vi "XImc Example One axis.vi"() -> ()   [LabVIEW 2012]
uses:
  subvi/XImc Example 1 CS.ctl
  libximc.lvlib
panel:
  in  "?":enum32{"Move settings"}(tab)
  in  "Speed":i32
  in  "GMOV":bool
  in  "SMOV":bool
  in  "Accel":i32
  in  "Decel":i32
  in  "Antiplay":i32
  out "Speed":dbl format="%#.2f"
  out "Accel":i16
  out "Decel":i16 format="%#.2f"
  out "Antiplay":i32
  out "Speed":dbl format="%#.2f steps/s"
  out "Temperature":dbl format="%#.2f C"
  out "USB current":dbl format="%#.2f mA"
  out "USB voltage":dbl format="%#.2f V"
  out "Power current":dbl format="%#.2f mA"
  out "Power voltage":dbl format="%#.2f V"
  in  "Stop motion":bool
  in  "ZEROCOMM":bool
  in  "HOME":bool
  in  "RIGHT":bool
  in  "LEFT":bool
  out "controller serial number":u32
  out "function return":i32
  out "Id":i32
  in  "SSTP":bool
  in  "Shift on":bool
  in  "?":i32
  in  "Move to":bool
  in  "?":i32
  out "?":dbl format="%#.2f"
  in  "Controller":u16(ring) items=["\\\\.\\COM7"]
  in  "Find controllers":bool
  in  "Close application":bool
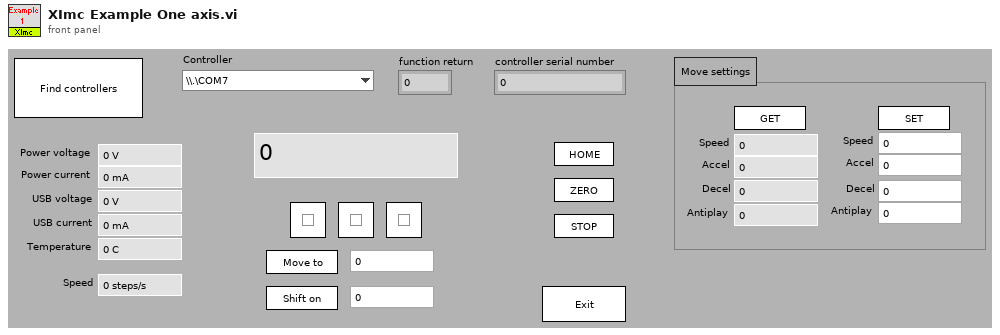
[diagram p1: front panel]
types:
  T1 = typedef "XImc Example 1 CS.ctl" = enum16{"Initialize_App", "Idle", "Find_Controllers", "Initialize_Controller", "Set_Parameters", "Get_Status", "Start_Motion", "Move_Relative", "Stop_Motion", "ZEROCOMM", "HOME", "LEFT", "RIGT", "SSTP", "Close_Controller", "Error_Handler", "Close_App", "Get_Move_Settings", "Set_Move_Settings"}
  T2 = cluster{"enumeration":i32, "Number of controllers":i32, "Controller name":string[], "variant":variant, "quit":bool, "Id":i32}
  T3 = cluster{"MoveSts":u32, "MvCmdSts":u32, "PWRSts":u32, "EncSts":u32, "WindSts":u32, "CurPosition":i32, "uCurPosition":i32, "@dummy control@":i8, "@dummy control@":i8, "@dummy control@":i8, "@dummy control@":i8, "EncPosition":i64, "CurSpeed":i32, "uCurSpeed":i32, "Ipwr":i32, "Upwr":i32, "Iusb":i32, "Uusb":i32, "CurT":i32, "Flags":u32, "GPIOFlags":u32, "CmdBufFreeSpace":u32}
  T4 = cluster{"Speed":u32, "uSpeed":u32, "Accel":u32, "Decel":u32, "AntiplaySpeed":u32, "uAntiplaySpeed":u32}
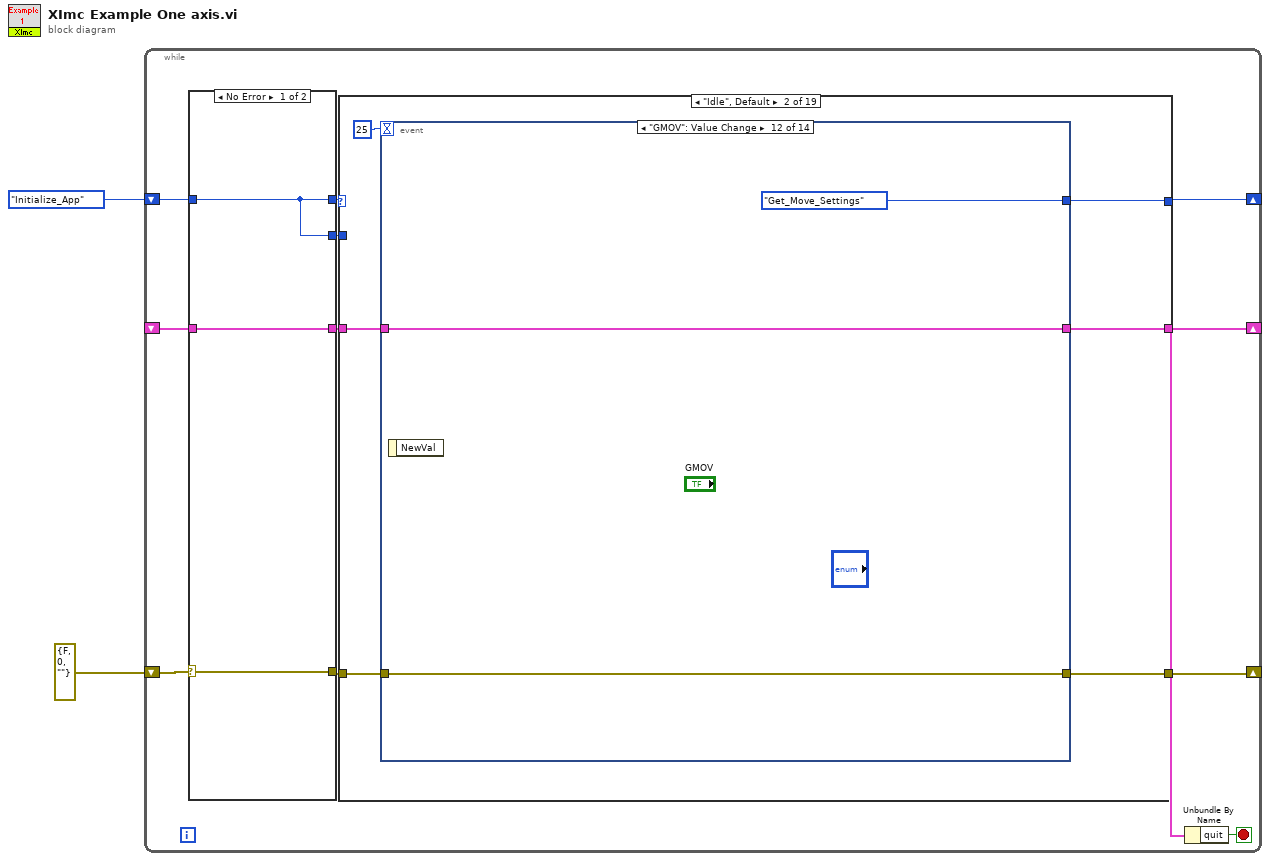
[diagram p0: block diagram]
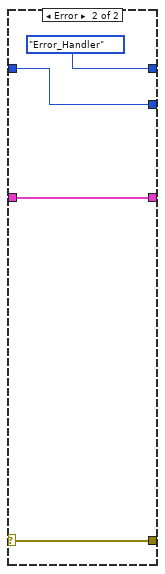
[diagram p2: hidden frame]
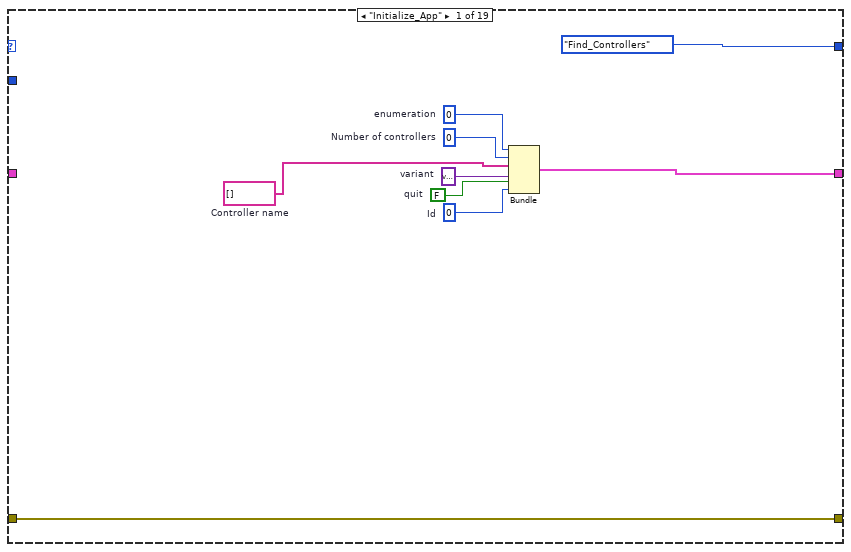
[diagram p3: hidden frame]
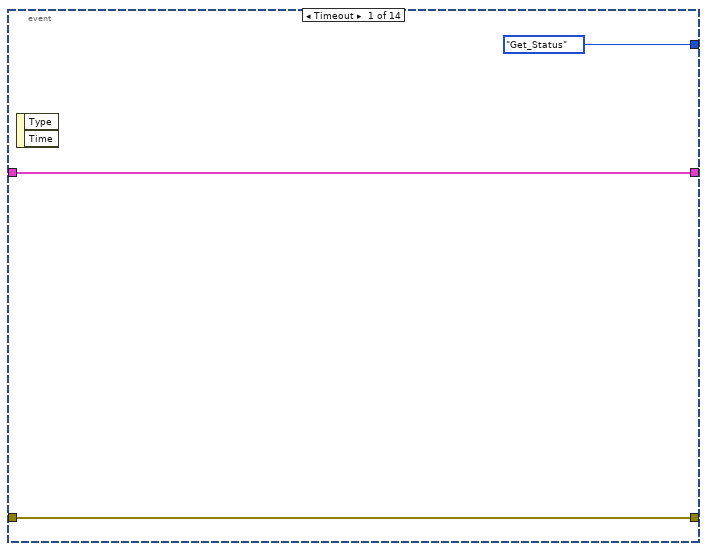
[diagram p4: hidden frame]
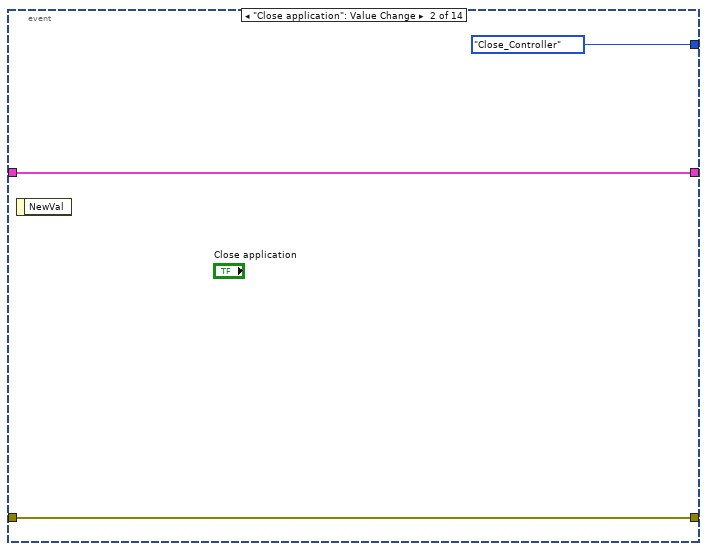
[diagram p5: hidden frame]
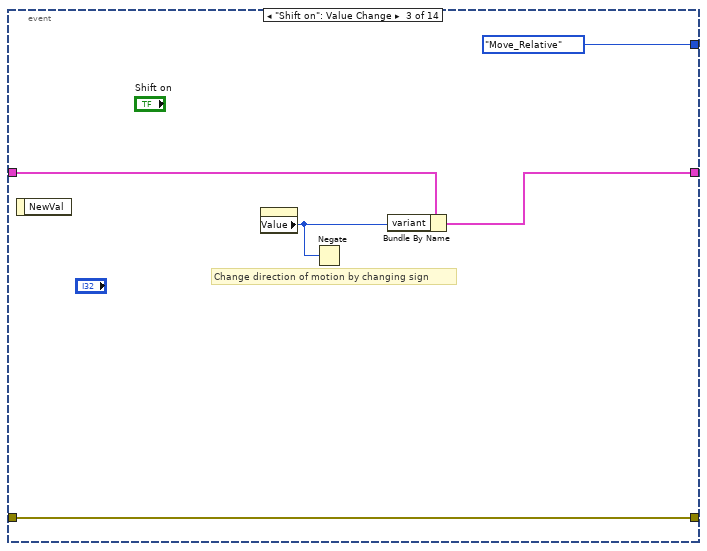
[diagram p6: hidden frame]
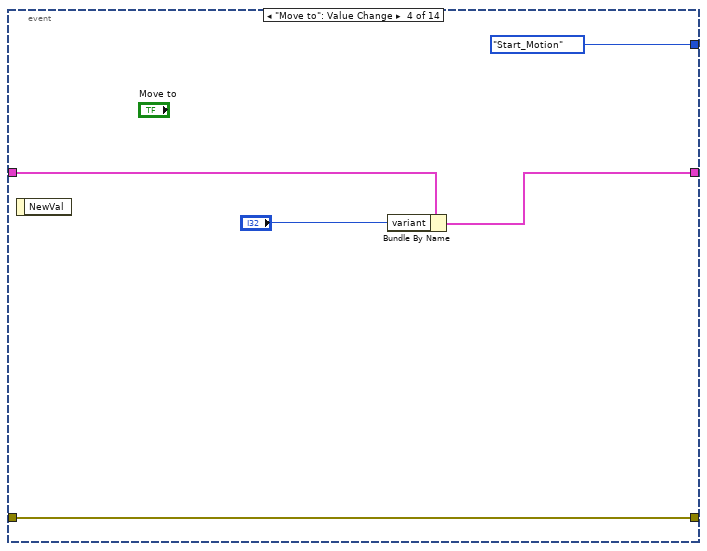
[diagram p7: hidden frame]
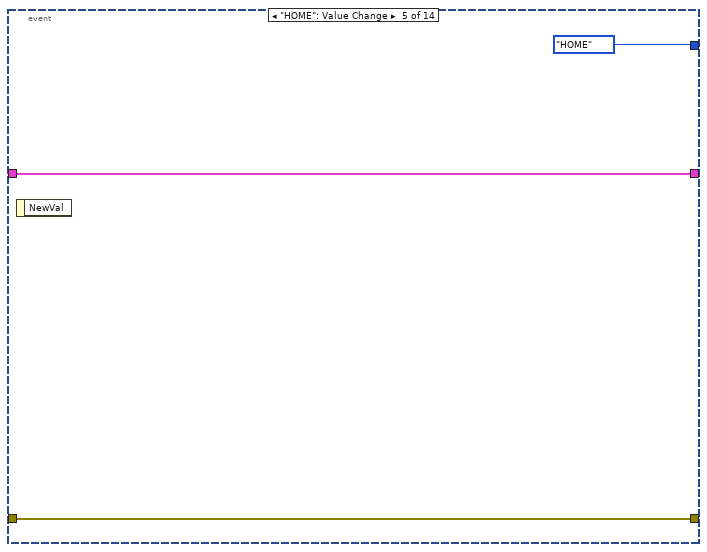
[diagram p8: hidden frame]
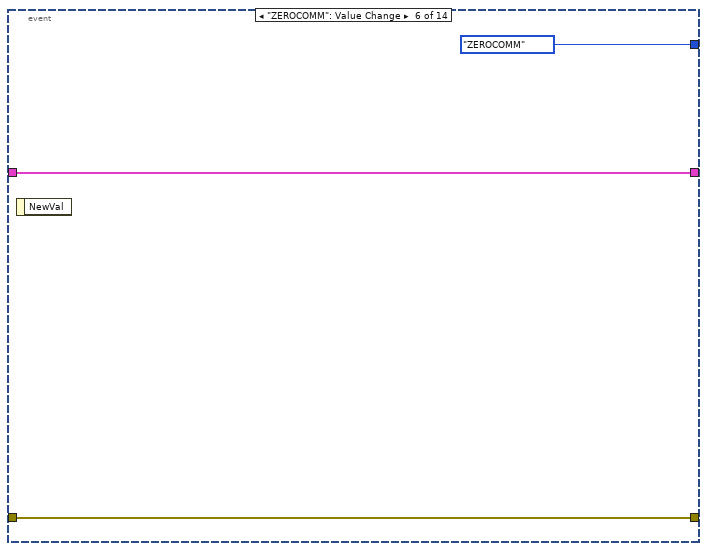
[diagram p9: hidden frame]
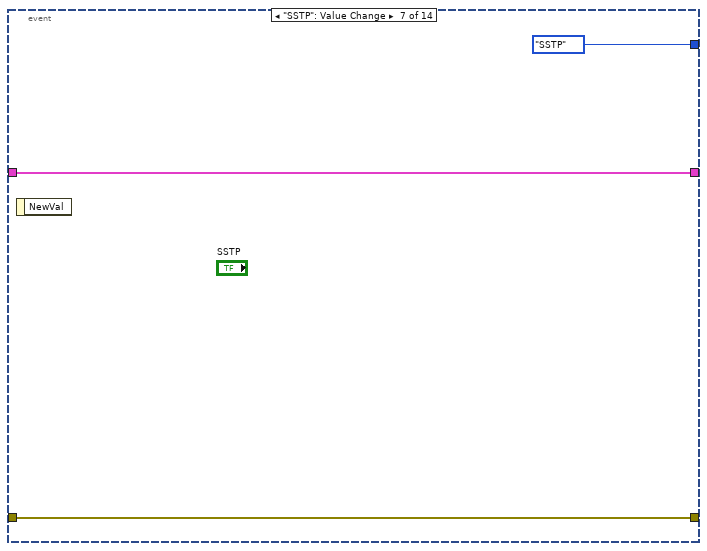
[diagram p10: hidden frame]
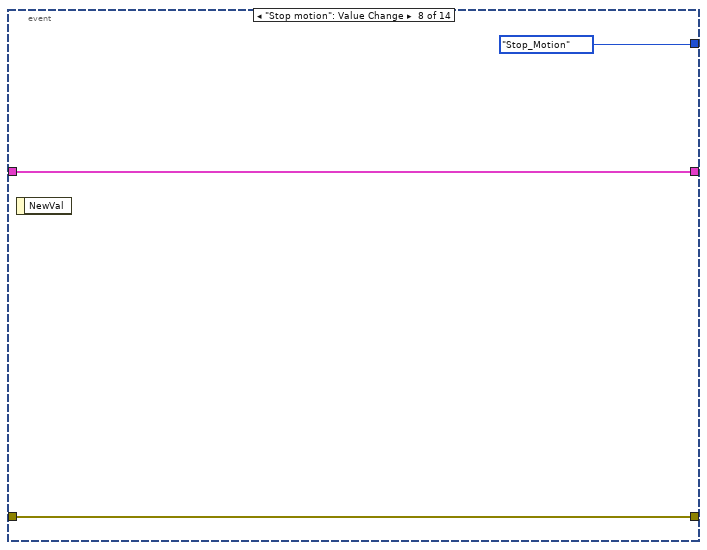
[diagram p11: hidden frame]
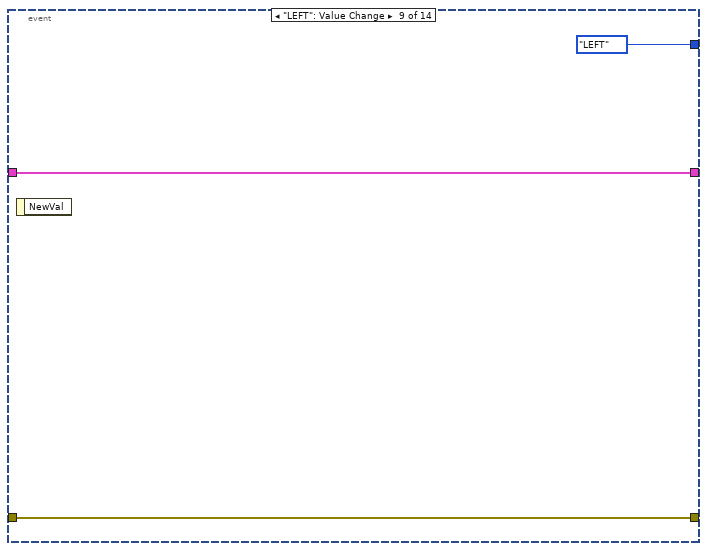
[diagram p12: hidden frame]
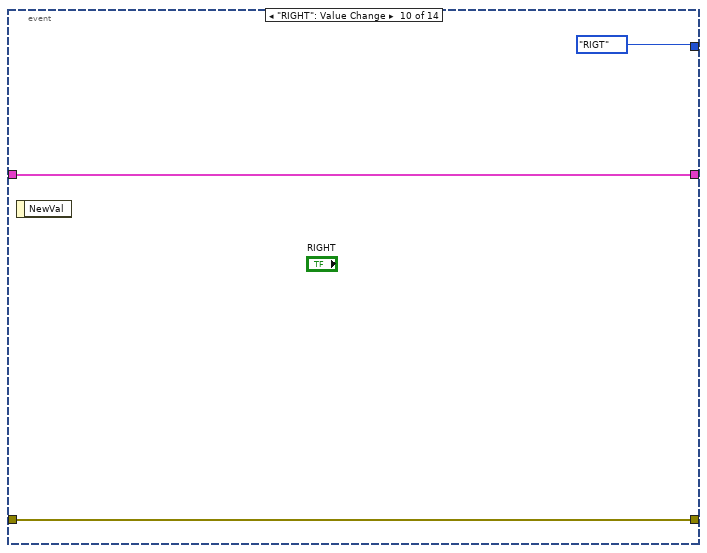
[diagram p13: hidden frame]
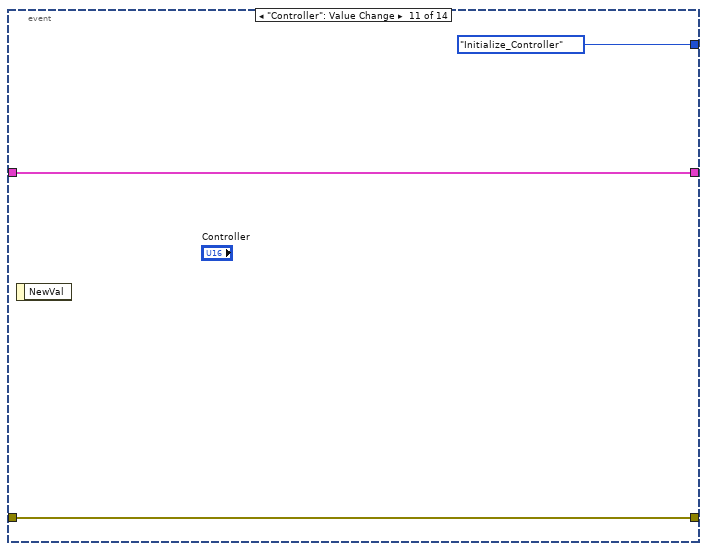
[diagram p14: hidden frame]
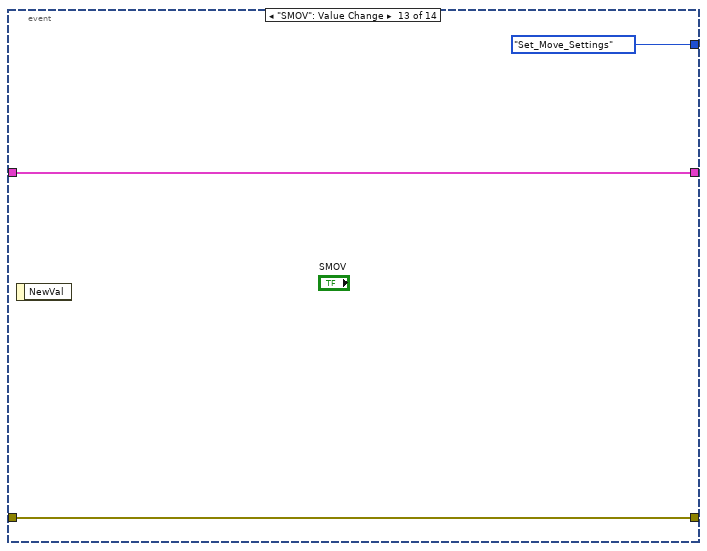
[diagram p15: hidden frame]
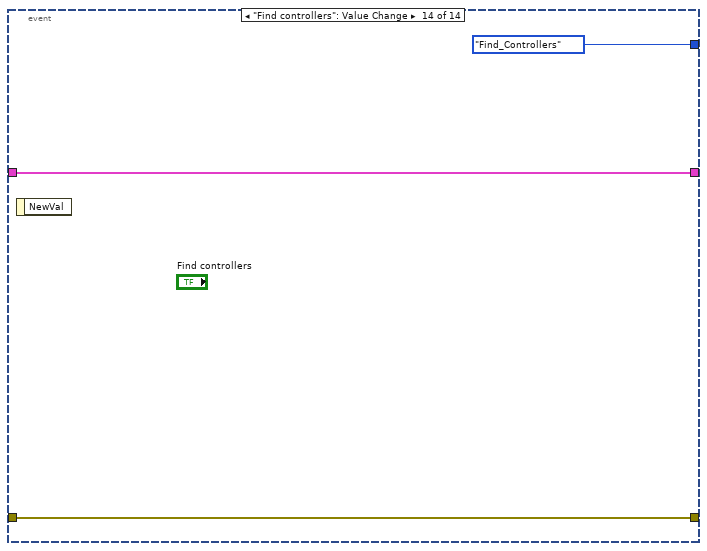
[diagram p16: hidden frame]
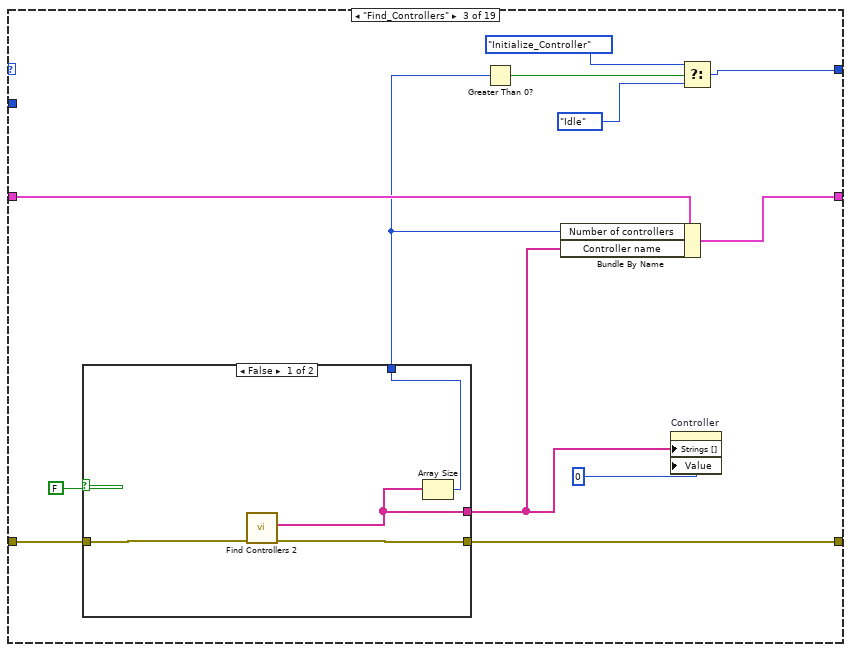
[diagram p17: hidden frame]
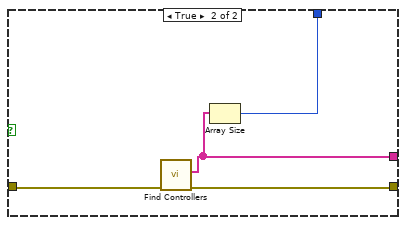
[diagram p18: hidden frame]
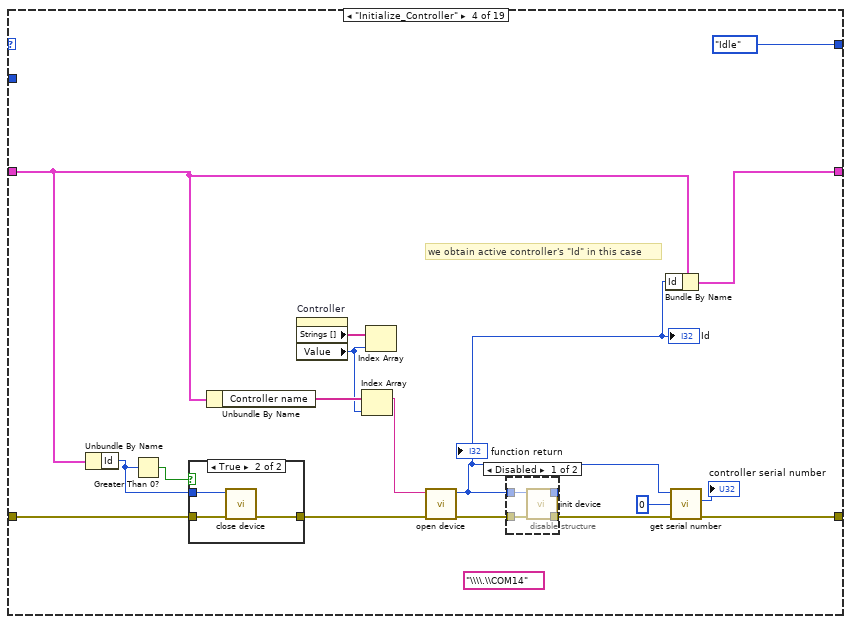
[diagram p19: hidden frame]
diagram:
  n1 = while {
    shift-right: [w13] -> _
    shift-left: XImc_Example_1_CS."Initialize_App" ("Case") -> [w6]
    shift-right: [w12] -> _
    shift-left: _ -> [w8]
    shift-right: [w3] -> _
    shift-left: errorcluster {"status"=FALSE, "code"=0, "source"=""} ("error in (no error)") -> [w10]
    stop <- w11 stop-if-true
    n2 = case shown="No Error" w10 {
      selector: w10 -> [w16 w19]
      tunnel: [w16 w19] -> w9
      tunnel: w8 -> [w15 w17]
      tunnel: [w15 w17] -> w7
      tunnel: w6 -> [w14 w18]
      tunnel: [w14 XImc_Example_1_CS."Error_Handler" ("Case")] -> w5
      tunnel: [w14 w18] -> w4
      frame No Error {
      }
      frame Error {
      }
    }
    n3 = case shown="\"Idle\", Default" w5 {
      tunnel: [XImc_Example_1_CS."Find_Controllers" ("Case") w33 w91 XImc_Example_1_CS."Idle" ("Case") XImc_Example_1_CS."Idle" ("Case") XImc_Example_1_CS."Idle" ("Case") XImc_Example_1_CS."Idle" ("Case") XImc_Example_1_CS."Idle" ("Case") XImc_Example_1_CS."Idle" ("Case") XImc_Example_1_CS."Idle" ("Case") XImc_Example_1_CS."Idle" ("Case") XImc_Example_1_CS."Idle" ("Case") XImc_Example_1_CS."Idle" ("Case") XImc_Example_1_CS."Idle" ("Case") XImc_Example_1_CS."Idle" ("Case") XImc_Example_1_CS."Idle" ("Case") XImc_Example_1_CS."Close_App" ("Case") w229 XImc_Example_1_CS."Idle" ("Case")] -> w13
      tunnel: [w26 w32 w88 w115 w128 w146 w156 w164 w169 w171 w179 w184 w186 w194 w196 w216 w221 w228 w231] -> w12
      tunnel: w9 -> [w25 w35 w87 w106 w127 w148 w153 w161 w168 w174 w177 w182 w188 w192 w201 w214 w219 w227 w234]
      tunnel: w7 -> [_ w31 w89 w108 w128 w146 w156 w164 w169 w171 w179 w184 w186 w194 w196 w216 w221 w228 w232]
      tunnel: w4 -> [_ _ _ _ _ _ _ _ _ _ _ _ _ _ _ _ _ w229 _]
      tunnel: [w25 w30 w86 w109 w127 w147 w152 w160 w166 w173 w176 w181 w187 w191 w203 w212 w222 w226 w234] -> w3
      frame "Initialize_App" {
        w21 = string[] []  # Controller name
        w22 = 0  # enumeration
        w23 = 0  # Number of controllers
        w24 = 0  # Id
        w27 = FALSE  # quit
        w28 = variant  # variant
        n4 = Bundle("enumeration"=w22, "Number of controllers"=w23, "Controller name"=w21, "variant"=w28, "quit"=w27, "Id"=w24) -> (w26:T2)  [unwired: 1 in]
      }
      frame "Idle", Default {
        n5 = event shown="[11] \"GMOV\": Value Change" {
          selector: _ -> [_ _ _ _ _ _ _ _ _ _ _ _ _ _]
          dyn-events: _ -> [_ _ _ _ _ _ _ _ _ _ _ _ _ _]
          timeout: 25 -> [_ _ _ _ _ _ _ _ _ _ _ _ _ _]
          tunnel: w35 -> [w36 w39 w45 w50 w53 w56 w59 w61 w65 w68 w71 w75 w76 w79]
          tunnel: [XImc_Example_1_CS."Get_Status" ("Case") XImc_Example_1_CS."Close_Controller" ("Case") XImc_Example_1_CS."Move_Relative" ("Case") XImc_Example_1_CS."Start_Motion" ("Case") XImc_Example_1_CS."HOME" ("Case") XImc_Example_1_CS."ZEROCOMM" ("Case") XImc_Example_1_CS."SSTP" ("Case") XImc_Example_1_CS."Stop_Motion" ("Case") XImc_Example_1_CS."LEFT" ("Case") XImc_Example_1_CS."RIGT" ("Case") XImc_Example_1_CS."Initialize_Controller" ("Case") XImc_Example_1_CS."Get_Move_Settings" ("Case") XImc_Example_1_CS."Set_Move_Settings" ("Case") XImc_Example_1_CS."Find_Controllers" ("Case")] -> w33
          tunnel: [w37 w40 w43 w48 w54 w57 w58 w62 w66 w69 w70 w73 w77 w80] -> w32
          tunnel: w31 -> [w37 w40 w44 w49 w54 w57 w58 w62 w66 w69 w70 w73 w77 w80]
          tunnel: [w36 w39 w45 w50 w53 w56 w59 w61 w65 w68 w71 w75 w76 w79] -> w30
          event Timeout {
            n6 = event-data() -> ()  [unwired: 1 in, 2 out]
          }
          event "Close application": Value Change {
            n7 = event-data() -> ()  [unwired: 1 in, 1 out]
          }
          event "Shift on": Value Change {
            # "Change direction of motion by changing sign"
            n8 = event-data() -> ()  [unwired: 1 in, 1 out]
            n9 = property class="DigNum (strict)"() -> ("Value"=w42:i32)  [unwired: 2 in, 2 out]
            n10 = Negate(x=w42) -> ()  [unwired: 1 out]
            n11 = Bundle By Name(cluster=w44, "variant"=w42) -> (w43:T2)
          }
          event "Move to": Value Change {
            n12 = event-data() -> ()  [unwired: 1 in, 1 out]
            n13 = Bundle By Name(cluster=w49, "variant"="?") -> (w48:T2)
          }
          event "HOME": Value Change {
            n14 = event-data() -> ()  [unwired: 1 in, 1 out]
          }
          event "ZEROCOMM": Value Change {
            n15 = event-data() -> ()  [unwired: 1 in, 1 out]
          }
          event "SSTP": Value Change {
            n16 = event-data() -> ()  [unwired: 1 in, 1 out]
          }
          event "Stop motion": Value Change {
            n17 = event-data() -> ()  [unwired: 1 in, 1 out]
          }
          event "LEFT": Value Change {
            n18 = event-data() -> ()  [unwired: 1 in, 1 out]
          }
          event "RIGHT": Value Change {
            n19 = event-data() -> ()  [unwired: 1 in, 1 out]
          }
          event "Controller": Value Change {
            n20 = event-data() -> ()  [unwired: 1 in, 1 out]
          }
          event "GMOV": Value Change {
            n21 = event-data() -> ()  [unwired: 1 in, 1 out]
          }
          event "SMOV": Value Change {
            n22 = event-data() -> ()  [unwired: 1 in, 1 out]
          }
          event "Find controllers": Value Change {
            n23 = event-data() -> ()  [unwired: 1 in, 1 out]
          }
        }
      }
      frame "Find_Controllers" {
        n24 = case shown="False" FALSE {
          tunnel: w87 -> [w96 w101]
          tunnel: [w97 w100] -> w86
          tunnel: [w94 w98] -> w85
          tunnel: [w95 w99] -> w82
          frame False {
            n25 = call "Find Controllers 2.vi"("error in (no error)"=w96) -> ("error out"=w97:errorcluster, "Names"=w95:string[])  [unwired: 9 in]
            n26 = Array Size(array=w95) -> (size(s)=w94:i32)
          }
          frame True {
            n27 = call "Find Controllers.vi"("error in (no error)"=w101) -> ("error out"=w100:errorcluster, "Controllers"=w99:string[])  [unwired: 8 in, 1 out]
            n28 = Array Size(array=w99) -> (size(s)=w98:i32)
          }
        }
        n29 = Greater Than 0?(x=w85) -> (x > 0?=w93:bool)
        n30 = Bundle By Name(cluster=w89, "Number of controllers"=w85, "Controller name"=w82) -> (w88:T2)
        n31 = property on="Controller" class="Ring (strict)"("Strings []"=w82, "Value"=0) -> ()  [unwired: 2 in, 2 out]
        n32 = Select(t=XImc_Example_1_CS."Initialize_Controller", s=w93, f=XImc_Example_1_CS."Idle" ("Case")) -> (s? t:f=w91:T1)
      }
      frame "Initialize_Controller" {
        (unwired) "\\\\.\\COM14" ("name")
        # "we obtain active controller's \"Id\" in this case"
        n33 = Unbundle By Name(w108) -> ("Id"=w107:i32)
        n34 = Greater Than 0?(x=w107) -> (x > 0?=w104:bool)
        n35 = case shown="True" w104 {
          tunnel: w107 -> [_ w122]
          tunnel: w106 -> [w119 w121]
          tunnel: [w119 w120] -> w105
          frame False {
          }
          frame True {
            n36 = call "close device.vi"("error in (no error)"=w121, "id"=w122) -> ("error out"=w120:errorcluster)  [unwired: 7 in, 2 out]
          }
        }
        n37 = Unbundle By Name(w108) -> ("Controller name"=w110:string[])
        n38 = property on="Controller" class="Ring (strict)"() -> ("Strings []"=w117:string[], "Value"=w102:u16)  [unwired: 2 in, 2 out]
        n39 = Index Array(array=w110, index=w102) -> (element=w103:string)
        n40 = Index Array(array=w117, index=w102) -> ()  [unwired: 1 out]
        n41 = call "open device.vi"("error in (no error)"=w105, "name"=w103) -> ("error out"=w116:errorcluster, "function return"=w111:i32)  [unwired: 8 in]
        "Id" <- w111
        "function return" <- w111
        n42 = disable-structure shown="Disabled" {
          disable-tunnel: w116 -> [w126 _]
          disable-tunnel: [w125 _] -> w113
          disable-tunnel: w111 -> [w124 _]
          disable-tunnel: [w123 _] -> _
          frame Disabled {
            n43 = call <userlib>:"init device.vi"("error in (no error)"=w126, "id"=w124) -> ("error out"=w125:errorcluster, "function return"=w123:i32)  [unwired: 8 in]
          }
          frame Enabled {
          }
        }
        n44 = Bundle By Name(cluster=w108, "Id"=w111) -> (w115:T2)
        n45 = call "get serial number.vi"("error in (no error)"=w113, "SerialNumber"=u32 0 ("serial"), "id"=w111) -> ("error out"=w109:errorcluster, "SerialNumber out"=→"controller serial number":u32)  [unwired: 6 in, 1 out]
      }
      frame "Set_Parameters" {
      }
      frame "Get_Status" {
        n46 = Unbundle By Name(w146) -> ("Id"=w145:i32)
        n47 = call "get status.vi"("error in (no error)"=w148, "id"=w145) -> ("error out"=w147:errorcluster, "status out"=w143:T3, "function return"=w144:i32)  [unwired: 7 in]
        n48 = Greater Or Equal To 0?(x=w144) -> ()  [unwired: 1 out]
        n49 = Unbundle By Name(w143) -> ("Upwr"=w138:i32, "Ipwr"=→"Power current":i32, "Uusb"=w136:i32, "Iusb"=→"USB current":i32, "CurT"=w132:i32, "CurSpeed"=→"Speed":i32, "CurPosition"=→"?":i32)  [unwired: 3 out]
        n50 = Multiply(x=0.01, y=w138) -> (x*y=→"Power voltage":dbl)
        n51 = Multiply(x=0.1, y=w132) -> (x*y=→"Temperature":dbl)
        n52 = Multiply(x=w136, y=0.01) -> (x*y=→"USB voltage":dbl)
      }
      frame "Start_Motion" {
        n53 = Unbundle By Name(w156) -> ("Id"=w150:i32, "variant"=w155:variant)
        n54 = Variant To Data(type=u32 0, Variant=w155) -> (data=w151:u32)  [unwired: 1 in, 1 out]
        n55 = call "command move.vi"("error in (no error)"=w153, "Position"=w151, "id"=w150) -> ("error out"=w152:errorcluster)  [unwired: 7 in, 1 out]
      }
      frame "Move_Relative" {
        n56 = Unbundle By Name(w164) -> ("Id"=w158:i32, "variant"=w163:variant)
        n57 = Variant To Data(type=0, Variant=w163) -> (data=w159:i32)  [unwired: 1 in, 1 out]
        n58 = call "command movr.vi"("error in (no error)"=w161, "DeltaPosition"=w159, "id"=w158) -> ("error out"=w160:errorcluster)  [unwired: 7 in, 1 out]
      }
      frame "Stop_Motion" {
        n59 = Unbundle By Name(w169) -> ("Id"=w167:i32)
        n60 = call "command stop.vi"("error in (no error)"=w168, "id"=w167) -> ("error out"=w166:errorcluster)  [unwired: 8 in, 1 out]
      }
      frame "SSTP" {
        n61 = Unbundle By Name(w171) -> ("Id"=w172:i32)
        n62 = call "command sstp.vi"("error in (no error)"=w174, "id"=w172) -> ("error out"=w173:errorcluster)  [unwired: 8 in, 1 out]
      }
      frame "LEFT" {
        n63 = Unbundle By Name(w179) -> ("Id"=w178:i32)
        n64 = call "command left.vi"("error in (no error)"=w177, "id"=w178) -> ("error out"=w176:errorcluster)  [unwired: 8 in, 1 out]
      }
      frame "RIGT" {
        n65 = Unbundle By Name(w184) -> ("Id"=w183:i32)
        n66 = call "command right.vi"("error in (no error)"=w182, "id"=w183) -> ("error out"=w181:errorcluster)  [unwired: 8 in, 1 out]
      }
      frame "HOME" {
        n67 = Unbundle By Name(w186) -> ("Id"=w189:i32)
        n68 = call "command home.vi"("error in (no error)"=w188, "id"=w189) -> ("error out"=w187:errorcluster)  [unwired: 8 in, 1 out]
      }
      frame "ZEROCOMM" {
        n69 = Unbundle By Name(w194) -> ("Id"=w193:i32)
        n70 = call "command zero.vi"("error in (no error)"=w192, "id"=w193) -> ("error out"=w191:errorcluster)  [unwired: 8 in, 1 out]
      }
      frame "Get_Move_Settings" {
        n71 = Unbundle By Name(w196) -> ("Id"=w204:i32)
        n72 = call "get move settings.vi"("error in (no error)"=w201, "id"=w204) -> ("error out"=w203:errorcluster, "move_settings out"=w202:T4)  [unwired: 7 in, 1 out]
        n73 = Unbundle By Name(w202) -> ("Speed"=→"Speed":u32, "Accel"=→"Accel":u32, "Decel"=→"Decel":u32, "AntiplaySpeed"=→"Antiplay":u32)  [unwired: 2 out]
      }
      frame "Set_Move_Settings" {
        n74 = call "get move settings.vi"() -> ("move_settings out"=w210:T4)  [unwired: 9 in, 2 out]
        n75 = Bundle(cluster=w210, "Speed"="Speed", "Accel"="Accel", "Decel"="Decel", "AntiplaySpeed"="Antiplay") -> (w211:T4)  [unwired: 2 in]
        n76 = Variant To Data(error in=w214, type=w210, Variant=w211) -> (data=w215:T4, error out=w213:errorcluster)
        n77 = Unbundle By Name(w216) -> ("Id"=w217:i32)
        n78 = call "set move settings.vi"("error in (no error)"=w213, "move_settings"=w215, "id"=w217) -> ("error out"=w212:errorcluster)  [unwired: 7 in, 1 out]
      }
      frame "Close_Controller" {
        n79 = Unbundle By Name(w221) -> ("Id"=w224:i32)
        n80 = call "close device.vi"("error in (no error)"=w219, "id"=w224) -> ("error out"=w223:errorcluster)  [unwired: 7 in, 2 out]
        n81 = Unbundle By Name(w221) -> ("enumeration"=w220:i32)  [unwired: 1 out]
        n82 = call "free enumerate devices.vi"("error in (no error)"=w223, "device_enumeration"=w220) -> ("error out"=w222:errorcluster)  [unwired: 8 in, 1 out]
      }
      frame "Error_Handler" {
        # "here we return to the last case before error occured"
        n83 = call <vilib>:"Clear Errors.vi"("error in (no error)"=w227) -> ("error out"=w226:errorcluster)  [unwired: 6 in]
      }
      frame "Close_App" {
        n84 = Bundle By Name(cluster=w232, "quit"=TRUE) -> (w231:T2)
      }
    }
    n85 = Unbundle By Name(w12) -> ("quit"=w11:bool)
  }
